vi "Consume Text.vi"(11 "Pattern Parser In":T1) -> (2 "Result":string, 3 "Pattern Parser":T1)   [LabVIEW 2020, in "Stream.lvlib" / "URLPattern.lvclass"]
uses:
  URLPattern.lvclass
  Token Type.ctl
  Token.ctl
  Pattern Part Type.ctl
  Pattern Part Modifier.ctl
  Pattern Part.ctl
  Pattern Parser.ctl
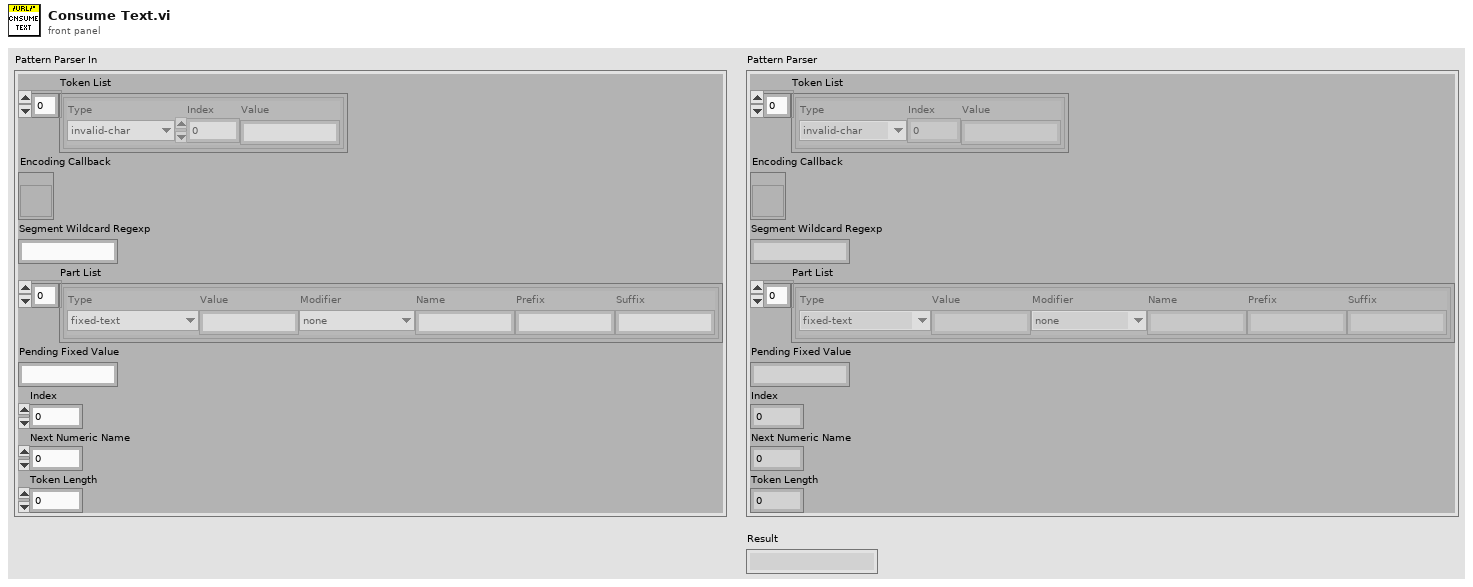
[diagram p1: front panel]
types:
  T1 = typedef "Stream.lvlib/URLPattern.lvclass/Pattern Parser.ctl" = cluster{"Token List":T2[], "Encoding Callback":refnum<vi>, "Segment Wildcard Regexp":string, "Part List":T4[], "Pending Fixed Value":string, "Index":i32, "Next Numeric Name":i32, "Token Length":i32}
  T2 = typedef "Stream.lvlib/URLPattern.lvclass/Token.ctl" = cluster{"Type":T3, "Index":i32, "Value":string}
  T3 = typedef "Stream.lvlib/URLPattern.lvclass/Token Type.ctl" = enum16{"invalid-char", "open", "close", "regexp", "name", "char", "escaped-char", "other-modifier", "asterisk", "end"}
  T4 = typedef "Stream.lvlib/URLPattern.lvclass/Pattern Part.ctl" = cluster{"Type":T5, "Value":string, "Modifier":T6, "Name":string, "Prefix":string, "Suffix":string}
  T5 = typedef "Stream.lvlib/URLPattern.lvclass/Pattern Part Type.ctl" = enum16{"fixed-text", "regexp", "segment-wildcard", "full-wildcard"}
  T6 = typedef "Stream.lvlib/URLPattern.lvclass/Pattern Part Modifier.ctl" = enum16{"none", "optional", "zero-or-more", "one-or-more"}
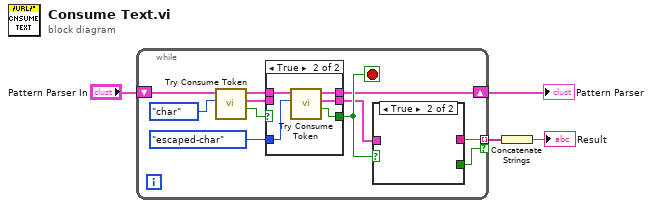
[diagram p0: block diagram]
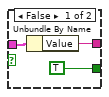
[diagram p2: hidden frame]
diagram:
  n1 = while {
    shift-right: [w7] -> w3
    shift-left: "Pattern Parser In" -> [w15]
    tunnel: [w6] -> w2 mode=indexing if=w5
    stop <- w9 stop-if-true
    n2 = call "Try Consume Token.vi"("Type"=Token_Type."char", "Pattern Parser In"=w15) -> ("Null?"=w11:bool, "Token"=w12:T2, "Pattern Parser"=w13:T1)  [unwired: 7 in]
    n3 = case shown="True" w11 {
      selector: w11 -> [w21 _]
      tunnel: w13 -> [w20 w26]
      tunnel: w12 -> [w19 _]
      tunnel: Token_Type."escaped-char" ("Type") -> [_ w25]
      tunnel: [w21 w24] -> w9
      tunnel: [w20 w22] -> w7
      tunnel: [w19 w23] -> w8
      frame False {
      }
      frame True {
        n4 = call "Try Consume Token.vi"("Type"=w25, "Pattern Parser In"=w26) -> ("Null?"=w24:bool, "Token"=w23:T2, "Pattern Parser"=w22:T1)  [unwired: 7 in]
      }
    }
    n5 = case shown="True" w9 {
      tunnel: w8 -> [w18 _]
      tunnel: [w17 _] -> w6
      tunnel: [TRUE _] -> w5
      frame False {
        n6 = Unbundle By Name(w18) -> ("Value"=w17:string)
      }
      frame True {
      }
    }
  }
  "Pattern Parser" <- w3
  n7 = Concatenate Strings(w2) -> (→"Result":string)
